vi "FIR2R.vi"(1 "FIR coefficients":dbl[](array[numeric])) -> (0 "Frequency":dbl[](array[numeric]))   [LabVIEW 2018]
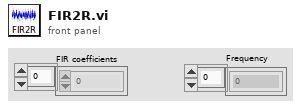
[diagram p1: front panel]
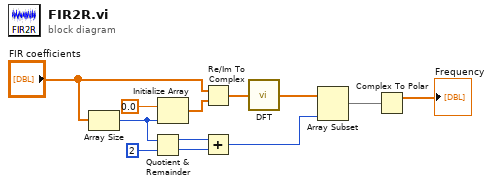
[diagram p0: block diagram]
diagram:
  n1 = Array Size(array="FIR coefficients") -> (size(s)=w2:i32)
  n2 = Quotient & Remainder(x=w2, y=2) -> (x-y*floor(x/y)=w11:i32, floor(x/y)=w10:i32)
  n3 = Initialize Array(0.0 ("element"), w2) -> (w8:dbl[])
  n4 = Re/Im To Complex(1:w8, 2:"FIR coefficients") -> (0:w6:cdb[])
  n5 = Add(x=w11, y=w10) -> (x+y=w1:i32)
  n6 = call "DFT.vi"("Input"=w6) -> ("Output"=w5:cdb[])
  n7 = Array Subset(array=w5, length=w1) -> (w4:cdb[])  [unwired: 1 in]
  n8 = Complex To Polar(r * e^(i*theta)=w4) -> (r=→"Frequency":dbl[])  [unwired: 1 out]
